vi "Read Shared Data DVR.vi"(8 "error in (no error)":errorcluster, 11 "Shared Data DVR in":T2) -> (0 "error out":errorcluster, 2 "shared data":T1, 3 "Shared Data DVR out":T2)   [LabVIEW 2017, in "DSF System Explorer.lvlib"]
uses:
  DSF System Explorer.lvlib
  shared data ref.ctl
  shared data.ctl
  DSF Core.lvlibp/Classes/Configuration/Configuration Session.lvclass
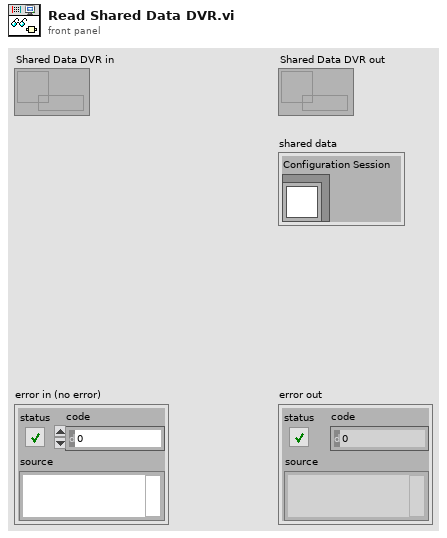
[diagram p1: front panel]
types:
  T1 = typedef "DSF System Explorer.lvlib/shared data.ctl" = cluster{"Configuration Session":refnum<class "Configuration Session.lvclass">}
  T2 = typedef "DSF System Explorer.lvlib/shared data ref.ctl" = refnum<data-value>
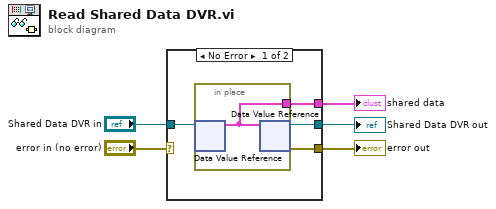
[diagram p0: block diagram]
diagram:
  n1 = case shown="No Error" "error in (no error)" {
    selector: "error in (no error)" -> [_ w11]
    tunnel: "Shared Data DVR in" -> [w9 w12]
    tunnel: [w8 _] -> w4
    tunnel: [w7 w12] -> w3
    tunnel: [w6 w11] -> w2
    frame No Error {
      n2 = in-place {
        in-place-border: [w10] -> w8
        n3 = in-place-dvr #1(w9) -> (w10:T1)  [unwired: 1 out]
        n4 = in-place-dvr #1(w10) -> (w7:T2, w6:errorcluster)
      }
    }
    frame Error {
    }
  }
  "error out" <- w2
  "Shared Data DVR out" <- w3
  "shared data" <- w4
